vi "TREE_tree header.vi"(7 "Direction":enum16{"READ", "WRITE"}(ring)=enum."WRITE", 8 "error in":errorcluster, 9 "Column Headers Visible (F)":bool, 10 "Column Header Strings":string[](array[string]), 11 "Tree In":refnum<vi>) -> (0 "error out":errorcluster, 2 "Column Header Strings out":string[](array[string]), 3 "Tree Out":refnum<vi>)   [LabVIEW 2011]
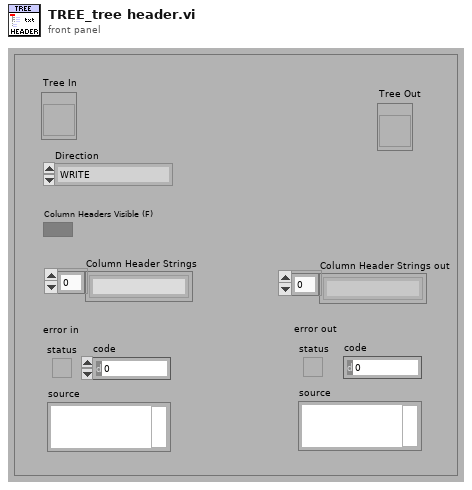
[diagram p1: front panel]
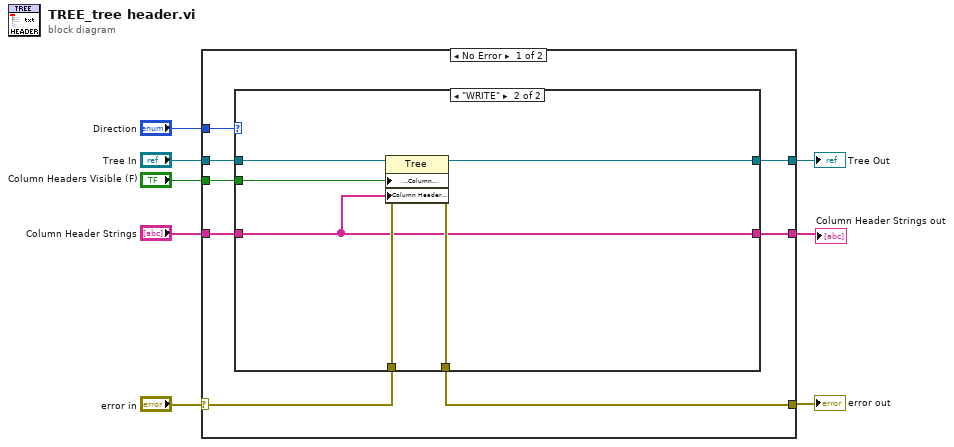
[diagram p0: block diagram]
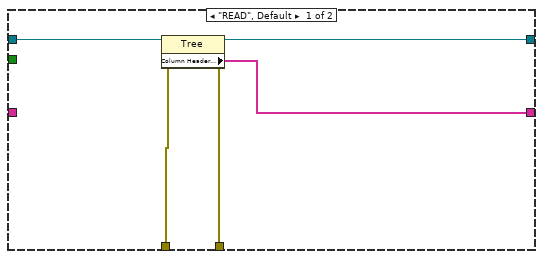
[diagram p2: hidden frame]
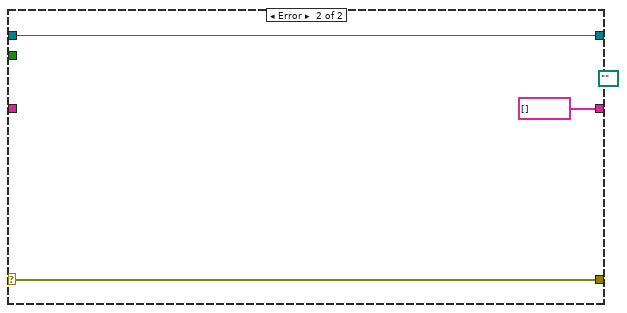
[diagram p3: hidden frame]
diagram:
  n1 = case shown="No Error" "error in" {
    selector: "error in" -> [w15 w29]
    tunnel: "Tree In" -> [w14 w28]
    tunnel: [w14 w28] -> w7
    tunnel: [w13 w29] -> w6
    tunnel: "Direction" -> [w12 _]
    tunnel: "Column Header Strings" -> [w11 _]
    tunnel: [w10 string[] [] ("directory names")] -> w2
    tunnel: "Column Headers Visible (F)" -> [w9 _]
    frame No Error {
      n2 = case shown="\"WRITE\"" w12 {
        tunnel: [w17 w26] -> _
        tunnel: w15 -> [w19 w25]
        tunnel: [w18 w24] -> w13
        tunnel: w14 -> [w20 w23]
        tunnel: w11 -> [_ w22]
        tunnel: [w16 w22] -> w10
        tunnel: w9 -> [_ w21]
        frame "READ", Default {
          n3 = property class="Tree"(reference=w20, error in=w19) -> (reference out=w17:refnum<vi>, error out=w18:errorcluster, "Column Header Strings[]"=w16:string[])
        }
        frame "WRITE" {
          n4 = property class="Tree"(reference=w23, error in=w25, "Visible Items:Column Headers Visible"=w21, "Column Header Strings[]"=w22) -> (reference out=w26:refnum<vi>, error out=w24:errorcluster)
        }
      }
    }
    frame Error {
      (unwired) path ""
      (unwired) "" ("name")
    }
  }
  "Tree Out" <- w7
  "error out" <- w6
  "Column Header Strings out" <- w2
